vi "Measurement Logic.vi"() -> ()   [LabVIEW 2021, in "adc_linearityMeasurement.lvlib"]
uses:
  adc_linearityMeasurement.lvlib
  <vilib>/DAQmx/create/channels.llb/DAQmx Create Channel (AO-Voltage-Basic).vi
  <resource>/objmgr/daqmx.rc
  <vilib>/gRPC/LabVIEW gRPC Library/Shared/grpcId.ctl
  <vilib>/gRPC/LabVIEW gRPC Library/grpc-lvsupport-release.lvlib
  shared/digitalInterface/client/dcvmDPI_AD7606B_clientImpl/dcvmDPI_AD7606B_clientImpl.lvlib
  shared/digitalInterface/client/dcvmDPI_AD7606B_client/dcvmDPI_AD7606B_client.lvlib
  <vilib>/DAQmx/configure/timing.llb/DAQmx Timing (Sample Clock).vi
  <vilib>/DAQmx/create/channels.llb/DAQmx Create Channel (AO-FuncGen).vi
  Measurement Configuration.ctl
  Measurement Results.ctl
  <vilib>/MeasurementLink/MeasurementLink Measurement Server/Classes/MeasurementContext/MeasurementContext.lvclass
panel:
  in  "Pin config":T1(array[cluster])=[{"Pin"="RESET", "Current Limit"=0.01, "Voltage Level"=3.3}, {"Pin"="SCLK", "Current Limit"=0.01, "Voltage Level"=3.3}, {"Pin"="CS", "Current Limit"=0.01, "Voltage Level"=3.3}, {"Pin"="WR", "Current Limit"=0.01, "Voltage Level"=3.3}, {"Pin"="CONVST", "Current Limit"=0.01, "Voltage Level"=0.0}, {"Pin"="REFSEL", "Current Limit"=0.01, "Voltage Level"=3.3}, {"Pin"="STBY", "Current Limit"=0.01, "Voltage Level"=3.3}, {"Pin"="SERPAR", "Current Limit"=0.01, "Voltage Level"=0.0}, {"Pin"="RANGE", "Current Limit"=0.01, "Voltage Level"=0.0}, {"Pin"="OS0", "Current Limit"=0.01, "Voltage Level"=0.0}, {"Pin"="OS1", "Current Limit"=0.01, "Voltage Level"=0.0}, {"Pin"="OS2", "Current Limit"=0.01, "Voltage Level"=0.0}, {"Pin"="RESET", "Current Limit"=0.01, "Voltage Level"=0.0}]
  out "Measurement Context out":refnum<class "MeasurementContext.lvclass">
  in  "Measurement Context":refnum<class "MeasurementContext.lvclass">
  out "Measurement Results":T2
  in  "Measurement Configuration":T3={"Input channel"=0, "Full scale range"=10.0, "Input signal"=0, "Analog source resource name"="", "Sine frequency"=1000.0, "Sine amplitude"=5.1, "Triangle frequency"=20.0, "Triangle amplitude"=5.1, "Ramp duration"=10.0, "Ramp amplitude"=5.05, "Ramp type"=0, "Digital capture resource name"="", "Digital capture sample rate"=800000.0, "Digital capture test duration"=800000.0} {"Ramp type" items=["Ascending", "Descending"]; "Input signal" items=["Sine", "Triangle", "Ramp"]}
  out "error out":errorcluster
  in  "error in":errorcluster
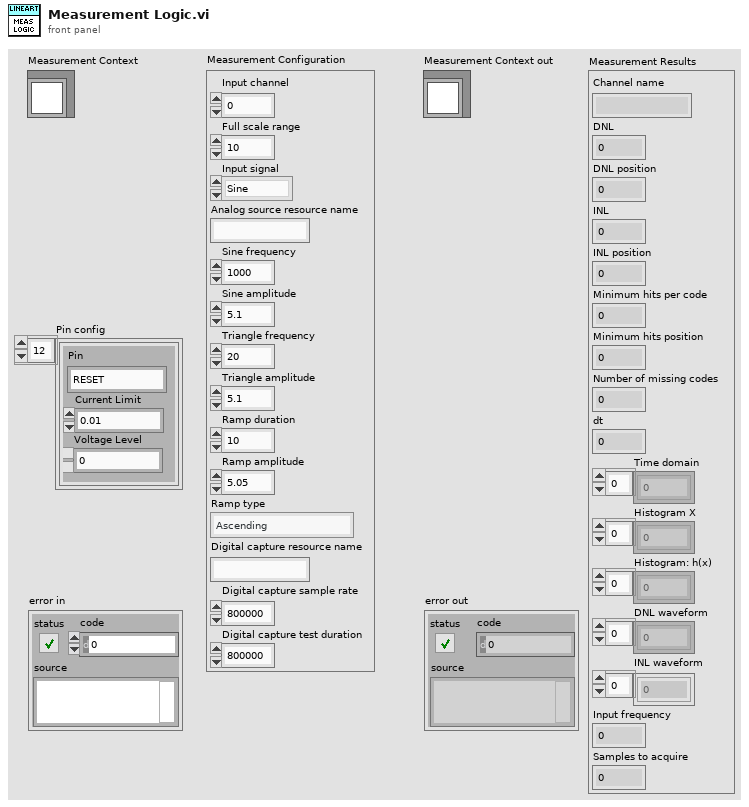
[diagram p1: front panel]
types:
  T1 = cluster{"Pin":string, "Current Limit":dbl, "Voltage Level":dbl}[]
  T2 = typedef "adc_linearityMeasurement.lvlib/Measurement Results.ctl" = cluster{"Channel name":string, "DNL":dbl, "DNL position":i32, "INL":dbl, "INL position":i32, "Minimum hits per code":i32, "Minimum hits position":i32, "Number of missing codes":i32, "dt":dbl, "Time domain":dbl[], "Histogram X":dbl[], "Histogram: h(x)":i32[], "DNL waveform":dbl[], "INL waveform":dbl[], "Input frequency":dbl, "Samples to acquire":u32}
  T3 = typedef "adc_linearityMeasurement.lvlib/Measurement Configuration.ctl" = cluster{"Input channel":i32, "Full scale range":dbl, "Input signal":u16, "Analog source resource name":string, "Sine frequency":dbl, "Sine amplitude":dbl, "Triangle frequency":dbl, "Triangle amplitude":dbl, "Ramp duration":dbl, "Ramp amplitude":dbl, "Ramp type":u16, "Digital capture resource name":string, "Digital capture sample rate":dbl, "Digital capture test duration":dbl}
  T4 = cluster{"Status":enum16{"NoAction", "GenerationStarted", "AcquisitionCompleted", "GenerationErrored"}, "Error":errorcluster}
  T5 = typedef "grpc-lvsupport-release.lvlib/grpcId.ctl" = u64
  T6 = cluster{"DSG Session":refnum<k21>, "gRPC session":T5, "Calculated frequency":dbl, "Calculated samples":u32, "DSG product name":string}
  T7 = enum16{"NoAction", "GenerationStarted", "AcquisitionCompleted", "GenerationErrored"}
  T8 = typedef "HW Sync Commands.ctl" = enum16{"NoAction", "GenerationStarted", "AcquisitionCompleted", "GenerationErrored"}
  T9 = cluster{"element":enum16{"NoAction", "GenerationStarted", "AcquisitionCompleted", "GenerationErrored"}, "error out":errorcluster}
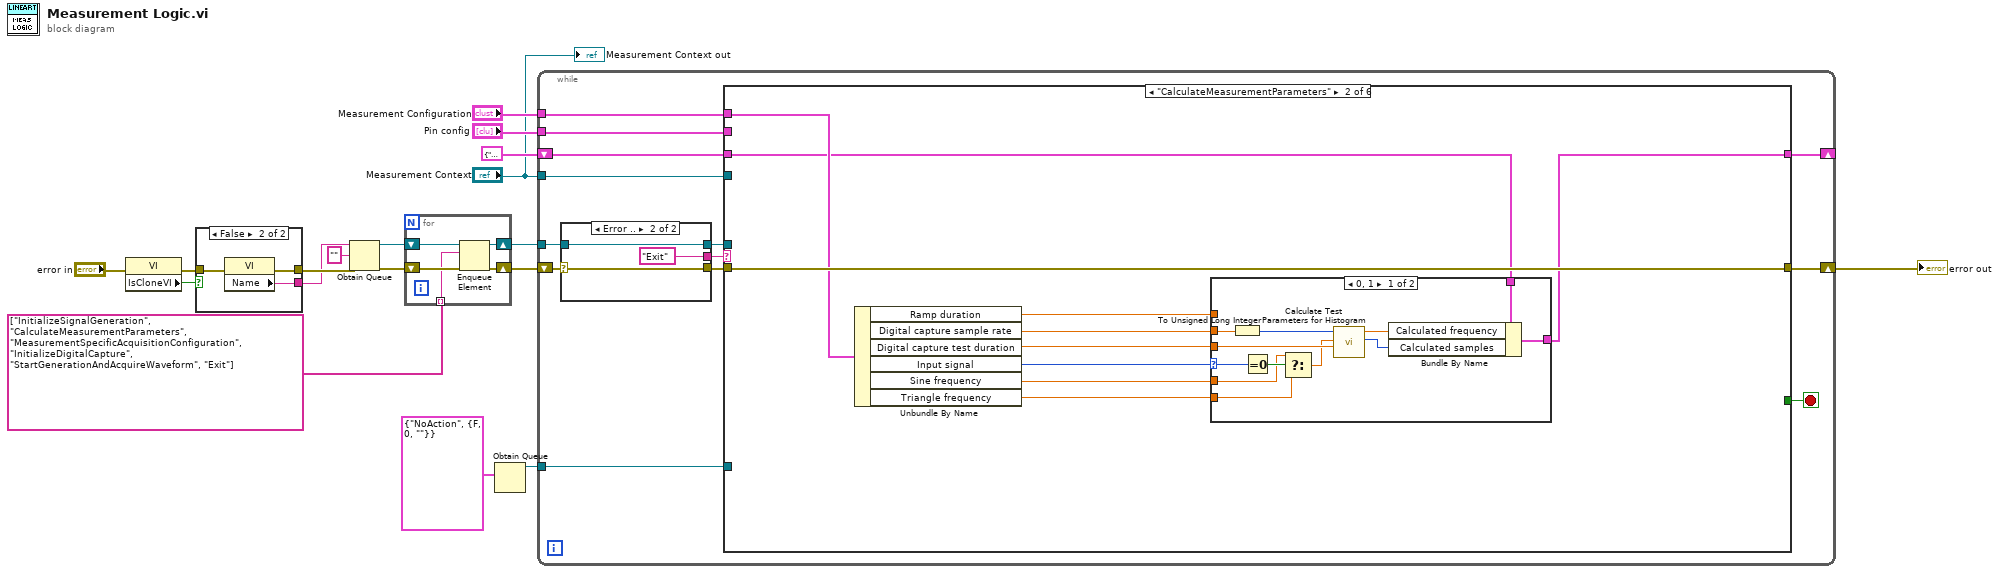
[diagram p0: block diagram]
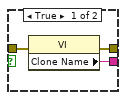
[diagram p2: hidden frame]
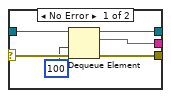
[diagram p3: hidden frame]
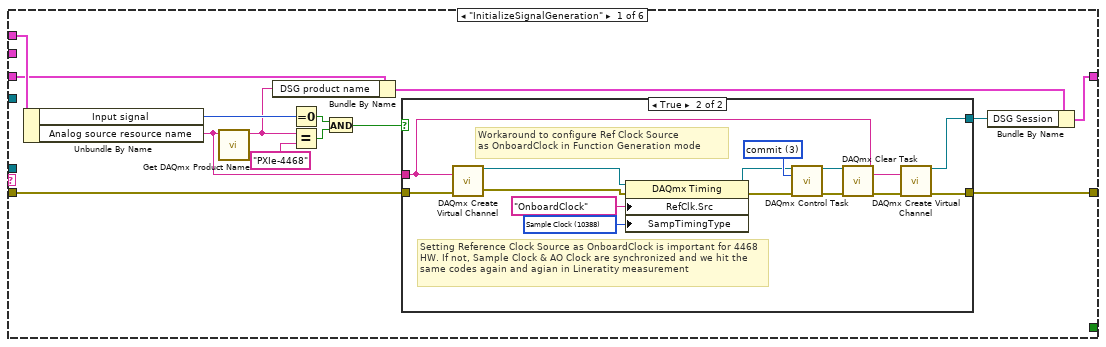
[diagram p4: hidden frame]
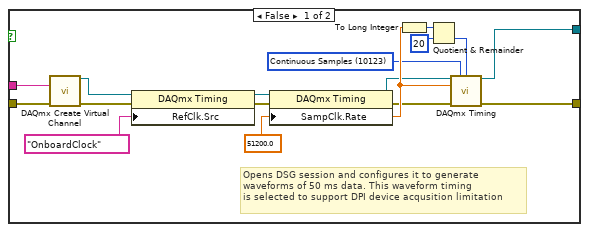
[diagram p5: hidden frame]
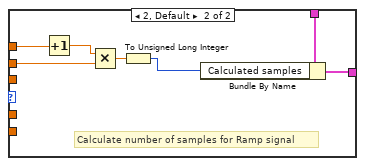
[diagram p6: hidden frame]
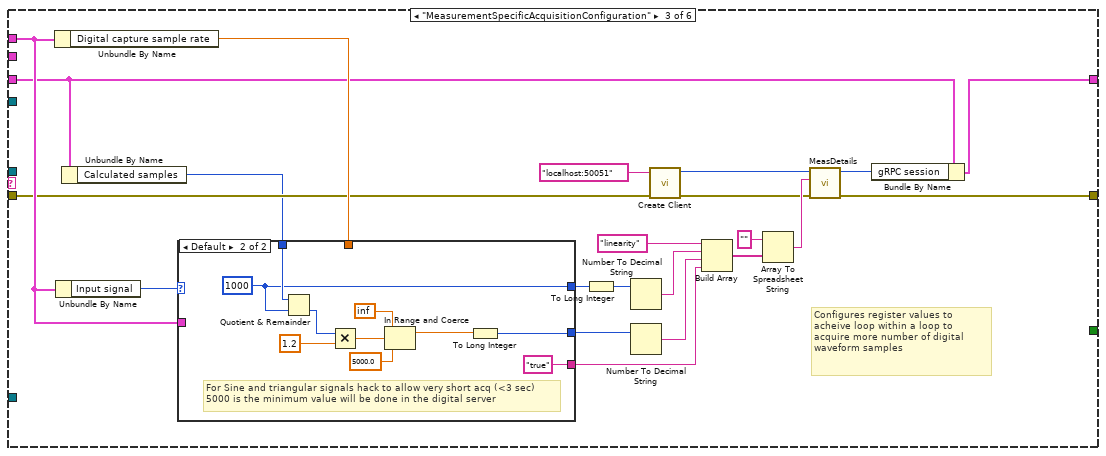
[diagram p7: hidden frame]
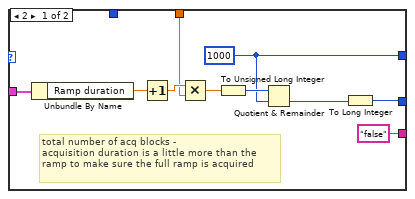
[diagram p8: hidden frame]
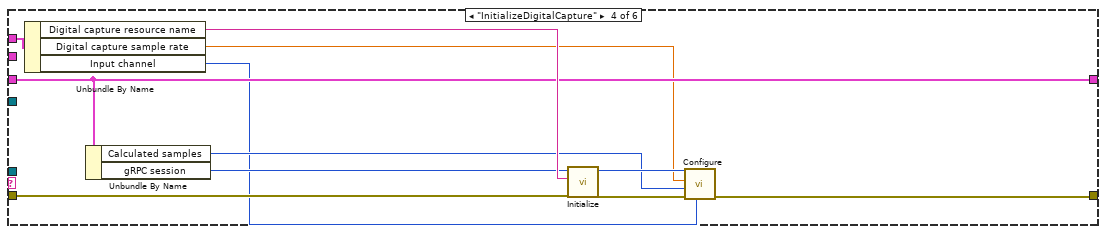
[diagram p9: hidden frame]
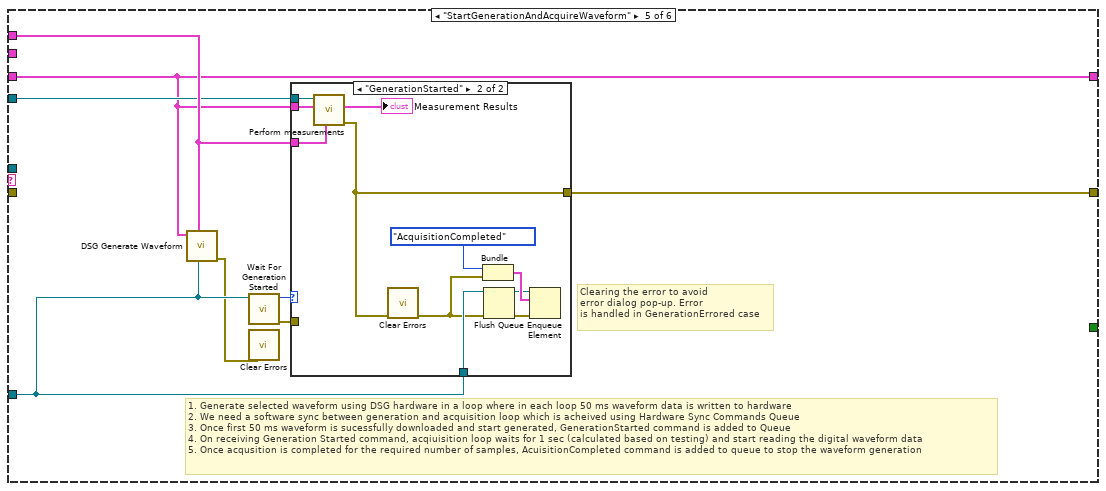
[diagram p10: hidden frame]
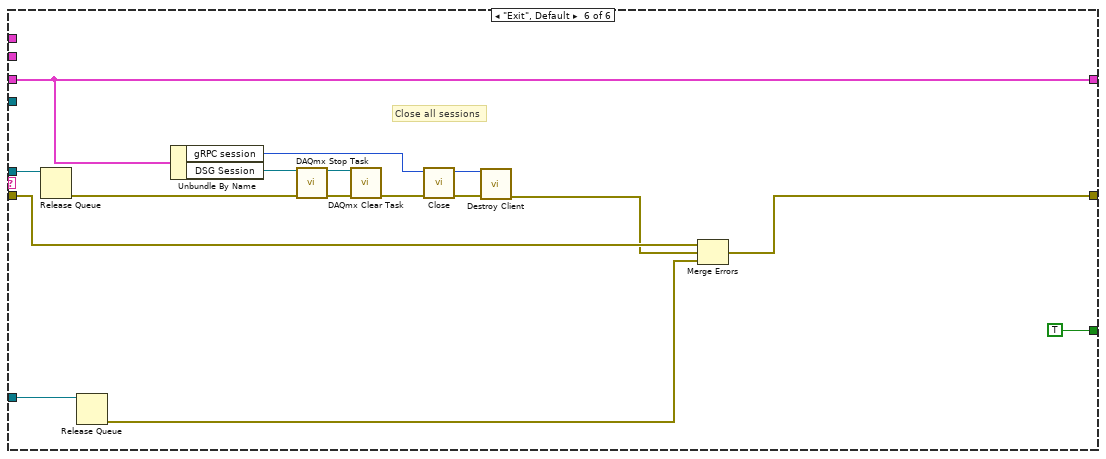
[diagram p12: hidden frame]
diagram:
  n1 = property class="VI"(error in="error in") -> (error out=w9:errorcluster, "IsCloneVI"=w10:bool)  [unwired: 1 in, 1 out]
  n2 = case shown="False" w10 {
    tunnel: [w21 w24] -> w8
    tunnel: [w20 w23] -> w7
    tunnel: w9 -> [w19 w22]
    frame True {
      n3 = property class="VI"(error in=w19) -> (error out=w21:errorcluster, "Clone Name"=w20:string)  [unwired: 1 in, 1 out]
    }
    frame False {
      n4 = property class="VI"(error in=w22) -> (error out=w24:errorcluster, "Name"=w23:string)  [unwired: 1 in, 1 out]
    }
  }
  n5 = Obtain Queue(name (unnamed)=w7, element data type="", error in (no error)=w8) -> (queue out=w17:refnum<queue>, error out=w6:errorcluster)  [unwired: 2 in, 1 out]
  n6 = for {
    shift-right: [w27] -> w16
    shift-left: w17 -> [w29]
    shift-right: [w26] -> w5
    shift-left: w6 -> [w28]
    tunnel: string[] ["InitializeSignalGeneration", "CalculateMeasurementParameters", "MeasurementSpecificAcquisitionConfiguration", "InitializeDigitalCapture", "StartGenerationAndAcquireWaveform", "Exit"] ("Step sequence") -> [w25] mode=indexing
    n7 = Enqueue Element(queue=w29, element=w25, error in (no error)=w28) -> (queue out=w27:refnum<queue>, error out=w26:errorcluster)  [unwired: 1 in, 1 out]
  }
  n8 = Obtain Queue(element data type=T4 {"Status"=enum."NoAction", "Error"={"status"=FALSE, "code"=0, "source"=""}}) -> (queue out=w12:refnum<queue>)  [unwired: 4 in, 2 out]
  n9 = while {
    tunnel: w16 -> [w34]
    shift-right: [w42] -> w2
    shift-left: w5 -> [w35]
    tunnel: "Measurement Configuration" -> [w40]
    shift-right: [w38] -> _
    shift-left: T6 {"DSG Session"="", "gRPC session"=0, "Calculated frequency"=0.0, "Calculated samples"=0, "DSG product name"=""} ("output cluster") -> [w39]
    tunnel: "Pin config" -> [w37]
    tunnel: w12 -> [w36]
    tunnel: "Measurement Context" -> [w30]
    stop <- w41 stop-if-true
    n10 = case shown="Error .." w35 {
      selector: w35 -> [w46 w50]
      tunnel: w34 -> [w48 w49]
      tunnel: [w47 "Exit" ("t")] -> w33
      tunnel: [w45 w50] -> w32
      tunnel: [w43 w49] -> w31
      frame No Error {
        n11 = Dequeue Element(queue=w48, timeout in ms (-1)=100, error in (no error)=w46) -> (queue out=w43:refnum<queue>, element=w47:string, error out=w45:errorcluster)  [unwired: 1 out]
      }
      frame Error {
      }
    }
    n12 = case shown="\"CalculateMeasurementParameters\"" w33 {
      tunnel: [w64 w105 w129 w170 w185 w204] -> w42
      tunnel: w32 -> [w65 w105 w142 w175 _ w205]
      tunnel: [_ _ _ _ _ TRUE] -> w41
      tunnel: w40 -> [w62 w104 w146 w177 w180 _]
      tunnel: w39 -> [w52 w97 w132 w174 w178 w209]
      tunnel: [w63 w98 w130 w174 w178 w209] -> w38
      tunnel: w37 -> [_ _ _ _ _ _]
      tunnel: w36 -> [_ _ _ _ w184 w208]
      tunnel: w31 -> [_ _ _ _ _ w207]
      tunnel: w30 -> [_ _ _ _ w179 _]
      frame "InitializeSignalGeneration" {
        n13 = Unbundle By Name(w62) -> ("Input signal"=w60:u16, "Analog source resource name"=w55:string)
        n14 = call "Get DAQmx Product Name.vi"("DAQmx resource name"=w55) -> ("DAQmx product type"=w54:string)  [unwired: 10 in]
        n15 = Bundle By Name(cluster=w52, "DSG product name"=w54) -> (w53:T6)
        n16 = Equal To 0?(x=w60) -> (x = 0?=w57:bool)
        n17 = Equal?(x=w54, y="PXIe-4468") -> (x = y?=w56:bool)
        n18 = And(x=w57, y=w56) -> (x .and. y?=w58:bool)
        n19 = case shown="True" w58 {
          tunnel: w55 -> [w81 w82]
          tunnel: w65 -> [w80 w85]
          tunnel: [w79 w84] -> w64
          tunnel: [w71 w83] -> w61
          frame False {
            w77 = 51200.0 ("SampClk.Rate")
            w72 = 10123 items=["Finite Samples"=10178, "Continuous Samples"=10123, "Hardware Timed Single Point"=12522] ("sample mode")
            # "Opens DSG session and configures it to generate\nwaveforms of 50 ms data. This waveform timing\nis selected to support DPI device acqusition limitation"
            n20 = call-poly <vilib>:"DAQmx Create Virtual Channel.vi"("physical channels"=w81, "error in"=w80) -> ("task out"=w68:refnum<k21>, "error out"=w69:errorcluster)  [unwired: 12 in]
            n21 = property class="DAQmx Timing"(reference=w68, error in=w69, "RefClk.Src"=tag "OnboardClock") -> (reference out=w67:refnum<k21>, error out=w66:errorcluster)
            n22 = property class="DAQmx Timing"(reference=w67, error in=w66, "SampClk.Rate"=w77) -> (reference out=w75:refnum<k21>, error out=w76:errorcluster)
            n23 = To Long Integer(number=w77) -> (32bit integer=w73:i32)
            n24 = Quotient & Remainder(x=w73, y=20) -> (floor(x/y)=w78:i32)  [unwired: 1 out]
            n25 = call-poly <vilib>:"DAQmx Timing.vi"("task/channels in"=w75, "sample mode"=w72, "samples per channel"=w78, "rate"=w77, "error in"=w76) -> ("task out"=w71:refnum<k21>, "error out"=w79:errorcluster)  [unwired: 9 in]
          }
          frame True {
            w86 = 10388 items=["Sample Clock"=10388, "Burst Handshake"=12548, "Handshake"=10389, "Implicit"=10451, "On Demand"=10390, "Change Detection"=12504, "Pipelined Sample Clock"=14668] ("SampTimingType")
            w92 = 3 items=["verify"=2, "reserve"=4, "commit"=3, "unreserve"=5, "abort"=6] ("action")
            # "Workaround to configure Ref Clock Source\nas OnboardClock in Function Generation mode"
            # "Setting Reference Clock Source as OnboardClock is important for 4468 HW. If not, Sample Clock & AO Clock are synchronized and we hit the same codes again and agian in Lineratity measurement"
            n26 = call-poly <vilib>:"DAQmx Create Virtual Channel.vi"("physical channels"=w82, "error in"=w85) -> ("task out"=w94:refnum<k21>, "error out"=w93:errorcluster)  [unwired: 12 in]
            n27 = property class="DAQmx Timing"(reference=w94, error in=w93, "RefClk.Src"=tag "OnboardClock", "SampTimingType"=w86) -> (reference out=w91:refnum<k21>, error out=w90:errorcluster)
            n28 = call <vilib>:"DAQmx Control Task.vi"("task/channels in"=w91, "action"=w92, "error in"=w90) -> ("task out"=w89:refnum<k21>, "error out"=w88:errorcluster)  [unwired: 11 in]
            n29 = call <vilib>:"DAQmx Clear Task.vi"("task in"=w89, "error in"=w88) -> ("error out"=w87:errorcluster)  [unwired: 13 in]
            n30 = call-poly <vilib>:"DAQmx Create Virtual Channel.vi"("physical channels"=w82, "error in"=w87) -> ("task out"=w83:refnum<k21>, "error out"=w84:errorcluster)  [unwired: 12 in]
          }
        }
        n31 = Bundle By Name(cluster=w53, "DSG Session"=w61) -> (w63:T6)
      }
      frame "CalculateMeasurementParameters" {
        n32 = Unbundle By Name(w104) -> ("Ramp duration"=w96:dbl, "Digital capture sample rate"=w102:dbl, "Digital capture test duration"=w101:dbl, "Input signal"=w103:u16, "Sine frequency"=w99:dbl, "Triangle frequency"=w100:dbl)
        n33 = case shown="0, 1" w103 {
          selector: w103 -> [w114 _]
          tunnel: w102 -> [w117 w124]
          tunnel: w101 -> [w115 _]
          tunnel: w100 -> [w112 _]
          tunnel: w99 -> [w111 _]
          tunnel: w97 -> [w109 w122]
          tunnel: [w107 w121] -> w98
          tunnel: w96 -> [_ w119]
          frame 0, 1 {
            n34 = To Unsigned Long Integer(number=w117) -> (unsigned 32bit integer=w116:u32)
            n35 = Equal To 0?(x=w114) -> (x = 0?=w113:bool)
            n36 = Select(t=w111, s=w113, f=w112) -> (s? t:f=w110:dbl)
            n37 = call "Calculate Test Parameters for Histogram.vi"("test duration (sec)"=w115, "input frequency"=w110, "sample rate"=w116) -> ("samples to acquire"=w106:u32, "input frequency"=w108:dbl)  [unwired: 5 in, 2 out]
            n38 = Bundle By Name(cluster=w109, "Calculated frequency"=w108, "Calculated samples"=w106) -> (w107:T6)
          }
          frame 2, Default {
            # "Calculate number of samples for Ramp signal"
            n39 = Increment(x=w119) -> (x+1=w118:dbl)
            n40 = Multiply(x=w118, y=w124) -> (x*y=w123:dbl)
            n41 = To Unsigned Long Integer(number=w123) -> (unsigned 32bit integer=w120:u32)
            n42 = Bundle By Name(cluster=w122, "Calculated samples"=w120) -> (w121:T6)
          }
        }
      }
      frame "MeasurementSpecificAcquisitionConfiguration" {
        # "Configures register values to acheive loop within a loop to acquire more number of digital waveform samples"
        n43 = Unbundle By Name(w146) -> ("Digital capture sample rate"=w144:dbl)
        n44 = Unbundle By Name(w146) -> ("Input signal"=w145:u16)
        n45 = Unbundle By Name(w132) -> ("Calculated samples"=w141:u32)
        n46 = case shown="Default" w145 {
          tunnel: w146 -> [w153 _]
          tunnel: [w152 w165] -> w128
          tunnel: [w148 w158] -> w126
          tunnel: w144 -> [w151 _]
          tunnel: w141 -> [_ w166]
          tunnel: ["false" "true"] -> w125
          frame 2 {
            w152 = u32 1000 ("value")
            # "total number of acq blocks -\nacquisition duration is a little more than the ramp to make sure the full ramp is acquired"
            n47 = Unbundle By Name(w153) -> ("Ramp duration"=w150:dbl)
            n48 = Increment(x=w150) -> (x+1=w154:dbl)
            n49 = Multiply(x=w154, y=w151) -> (x*y=w156:dbl)
            n50 = To Unsigned Long Integer(number=w156) -> (unsigned 32bit integer=w155:u32)
            n51 = Quotient & Remainder(x=w155, y=w152) -> (floor(x/y)=w149:u32)  [unwired: 1 out]
            n52 = To Long Integer(number=w149) -> (32bit integer=w148:i32)
          }
          frame Default {
            w165 = u32 1000 ("value")
            # "For Sine and triangular signals hack to allow very short acq (<3 sec)\n5000 is the minimum value will be done in the digital server"
            n53 = Quotient & Remainder(x=w166, y=w165) -> (floor(x/y)=w164:u32)  [unwired: 1 out]
            n54 = Multiply(x=w164, y=1.2) -> (x*y=w162:dbl)
            n55 = In Range and Coerce(upper limit=inf, x=w162, lower limit=5000.0) -> (coerced(x)=w159:dbl)  [unwired: 1 out]
            n56 = To Long Integer(number=w159) -> (32bit integer=w158:i32)
          }
        }
        n57 = To Long Integer(number=w128) -> (32bit integer=w127:i32)
        n58 = Number To Decimal String(number=w127) -> (decimal integer string=w139:string)  [unwired: 1 in]
        n59 = Number To Decimal String(number=w126) -> (decimal integer string=w138:string)  [unwired: 1 in]
        n60 = call "Create Client.vi"("error in"=w142, "address"="localhost:50051") -> ("error out"=w133:errorcluster, "gRPC ID Out"=w135:T5)  [unwired: 8 in]
        n61 = Build Array("linearity", w139, w138, w125) -> (w137:string[])
        n62 = Array To Spreadsheet String(array=w137, 3:"" ("format string")) -> (spreadsheet string=w134:string)  [unwired: 1 in]
        n63 = call "MeasDetails.vi"("error in"=w133, "Active measurement"=w134, "gRPC session in"=w135) -> ("error out"=w129:errorcluster, "gRPC session out"=w131:T5)  [unwired: 7 in]
        n64 = Bundle By Name(cluster=w132, "gRPC session"=w131) -> (w130:T6)
      }
      frame "InitializeDigitalCapture" {
        n65 = Unbundle By Name(w177) -> ("Digital capture resource name"=w176:string, "Digital capture sample rate"=w169:dbl, "Input channel"=w167:i32)
        n66 = Unbundle By Name(w174) -> ("Calculated samples"=w168:u32, "gRPC session"=w173:T5)
        n67 = call "Initialize.vi"("error in"=w175, "Digital capture resource name"=w176, "gRPC session in"=w173) -> ("error out"=w171:errorcluster, "gRPC session out"=w172:T5)  [unwired: 7 in]
        n68 = call "Configure.vi"("Input channel"=w167, "error in"=w171, "Digital capture samples"=w168, "Digital capture sample rate"=w169, "gRPC session in"=w172) -> ("error out"=w170:errorcluster)  [unwired: 5 in, 1 out]
      }
      frame "StartGenerationAndAcquireWaveform" {
        # "1. Generate selected waveform using DSG hardware in a loop where in each loop 50 ms waveform data is written to hardware\n2. We need a software sync between generation and acquisition loop which is acheived using Hardware Sync Commands Queue\n3. Once first 50 ms waveform is sucessfully downloaded and start generated, GenerationStarted command is added to Queue\n4. On receiving Generation Started command, acqiuisition loop waits for 1 sec (calculated based on testing) and start reading the digital waveform data\n5. Once acqusition is completed for the required number of samples, AcuisitionCompleted command is added to queue to stop the waveform generation"
        # "Clearing the error to avoid\nerror dialog pop-up. Error\nis handled in GenerationErrored case"
        n69 = call "DSG Generate Waveform.vi"("hardware sync commands queue"=w184, "measurement configuration"=w180, "meas logic calculated values"=w178) -> ("error out"=w181:errorcluster)  [unwired: 7 in, 1 out]
        n70 = call "Wait For Generation Started.vi"("hardware commands sync queue"=w184) -> ("error out"=w182:errorcluster, "Status"=w183:T8)  [unwired: 9 in]
        n71 = call <vilib>:"Clear Errors.vi"("error in (no error)"=w181) -> ()  [unwired: 5 in, 2 out]
        n72 = case shown="\"GenerationStarted\"" w183 {
          tunnel: [w186 w187] -> w185
          tunnel: w184 -> [_ w194]
          tunnel: w178 -> [_ w190]
          tunnel: w180 -> [_ w189]
          tunnel: w182 -> [w186 _]
          tunnel: w179 -> [_ w191]
          frame Default {
          }
          frame "GenerationStarted" {
            n73 = call "Perform measurements.vi"("measurement configuration"=w189, "meas logic calculated values"=w190, "measurement context in"=w191) -> ("error out"=w187:errorcluster, "measurement results"=→"Measurement Results":T2)  [unwired: 7 in]
            n74 = call <vilib>:"Clear Errors.vi"("error in (no error)"=w187) -> ("error out"=w193:errorcluster)  [unwired: 5 in, 1 out]
            n75 = Bundle("element"=T7."AcquisitionCompleted", "error out"=w193) -> (w196:T9)  [unwired: 1 in]
            n76 = Flush Queue(queue=w194, error in (no error)=w193) -> (queue out=w195:refnum<queue>, error out=w192:errorcluster)  [unwired: 1 out]
            n77 = Enqueue Element(queue=w195, element=w196, error in (no error)=w192) -> ()  [unwired: 1 in, 3 out]
          }
        }
      }
      frame "Exit", Default {
        # "Close all sessions"
        n78 = Release Queue(queue=w207) -> (error out=w206:errorcluster)  [unwired: 2 in, 2 out]
        n79 = Release Queue(queue=w208) -> (error out=w203:errorcluster)  [unwired: 2 in, 2 out]
        n80 = Unbundle By Name(w209) -> ("gRPC session"=w202:T5, "DSG Session"=w212:refnum<k21>)
        n81 = call <vilib>:"DAQmx Stop Task.vi"("task/channels in"=w212, "error in"=w206) -> ("task out"=w211:refnum<k21>, "error out"=w210:errorcluster)  [unwired: 12 in]
        n82 = call <vilib>:"DAQmx Clear Task.vi"("task in"=w211, "error in"=w210) -> ("error out"=w201:errorcluster)  [unwired: 13 in]
        n83 = call "Close.vi"("error in"=w201, "gRPC session in"=w202) -> ("error out"=w199:errorcluster, "gRPC session out"=w200:T5)  [unwired: 8 in]
        n84 = call "Destroy Client.vi"("error in"=w199, "gRPC ID"=w200) -> ("error out"=w198:errorcluster)  [unwired: 9 in]
        n85 = Merge Errors(w205, w198, w203) -> (w204:errorcluster)
      }
    }
  }
  "error out" <- w2
  "Measurement Context out" <- "Measurement Context"
